vi "TR_Generate_Segmented_Plot_v5_DAQmx.vi"(0 "Settings and Parameters in":T1, 1 "Background color":u32(colorbox)=13816530, 2 "Segments Colors In":T6={"Colors array for outer segments"=[14102567, 16625249, 14742520, 7646673, 16018755, 16703632, 11262441, 4552116], "Colors array for midfield segments"=[8073876, 10935200, 34871, 12756431], "Color for central segment"=16777113, "Fill color for no segments image"=6316128}, 3 "Scale factor for outer display radius display (0.95)":dbl=0.95 format="%#_13g", 5 "Regions to mark set/selected":T4, 7 "Show magnets (T)":bool=TRUE, 9 "Show zones (T)":bool=TRUE, 11 "Error In":errorcluster) -> (4 "Settings and Parameters out":T1, 6 "Experiment Diagram":T7(plugin-control), 8 "Color to [pixel, segment, zone] correspondences":T3, 10 "Image geometrical and scaling parameters":T5, 15 "Error Out":errorcluster)   [LabVIEW 2018, in "Tracks Repair.lvlib"]
uses:
  Tracks Repair.lvlib
  SubVi's/Controls/CTL_Image_Geometrical_and_scaling_parameters.ctl
  SubVi's/Controls/CTL_Pixel_to_Zone_array.ctl
  SubVi's/Controls/CTL_Settings_cluster.ctl
  SubVi's/Controls/CTL_Histogram_parameters.ctl
  SubVi's/Controls/CTL_Filter_selector.ctl
  SubVi's/Controls/CTL_Acquisition_speed_selector.ctl
  SubVi's/Controls/CTL_Segmented_plot_parameters.ctl
  SubVi's/Controls/CTL_IO_params_cluster.ctl
  SubVi's/Controls/CTL_Conditions_Array.ctl
  SubVi's/Controls/CTL_Conditions_Cluster.ctl
  SubVi's/Controls/CTL_Condition_type.ctl
  SubVi's/Controls/CTL_Comparison_type.ctl
  SubVi's/Controls/CTL_Validity_check_criteria.ctl
  SubVi's/Controls/CTL_Response_info.ctl
  SubVi's/Controls/CTL_Condition_response_type.ctl
  SubVi's/Controls/CTL_Reponse_port_info.ctl
  SubVi's/Controls/CTL_Calibration_parameters.ctl
  SubVi's/Controls/CTL_Dispenser_calibration_info.ctl
  SubVi's/Controls/CTL_Post-processing_params.ctl
  SubVi's/Controls/CTL_Mouse_Draw_Params.ctl
  <vilib>/vision/Image Controls.llb/IMAQ Image.ctl
  Tracker.lvlib
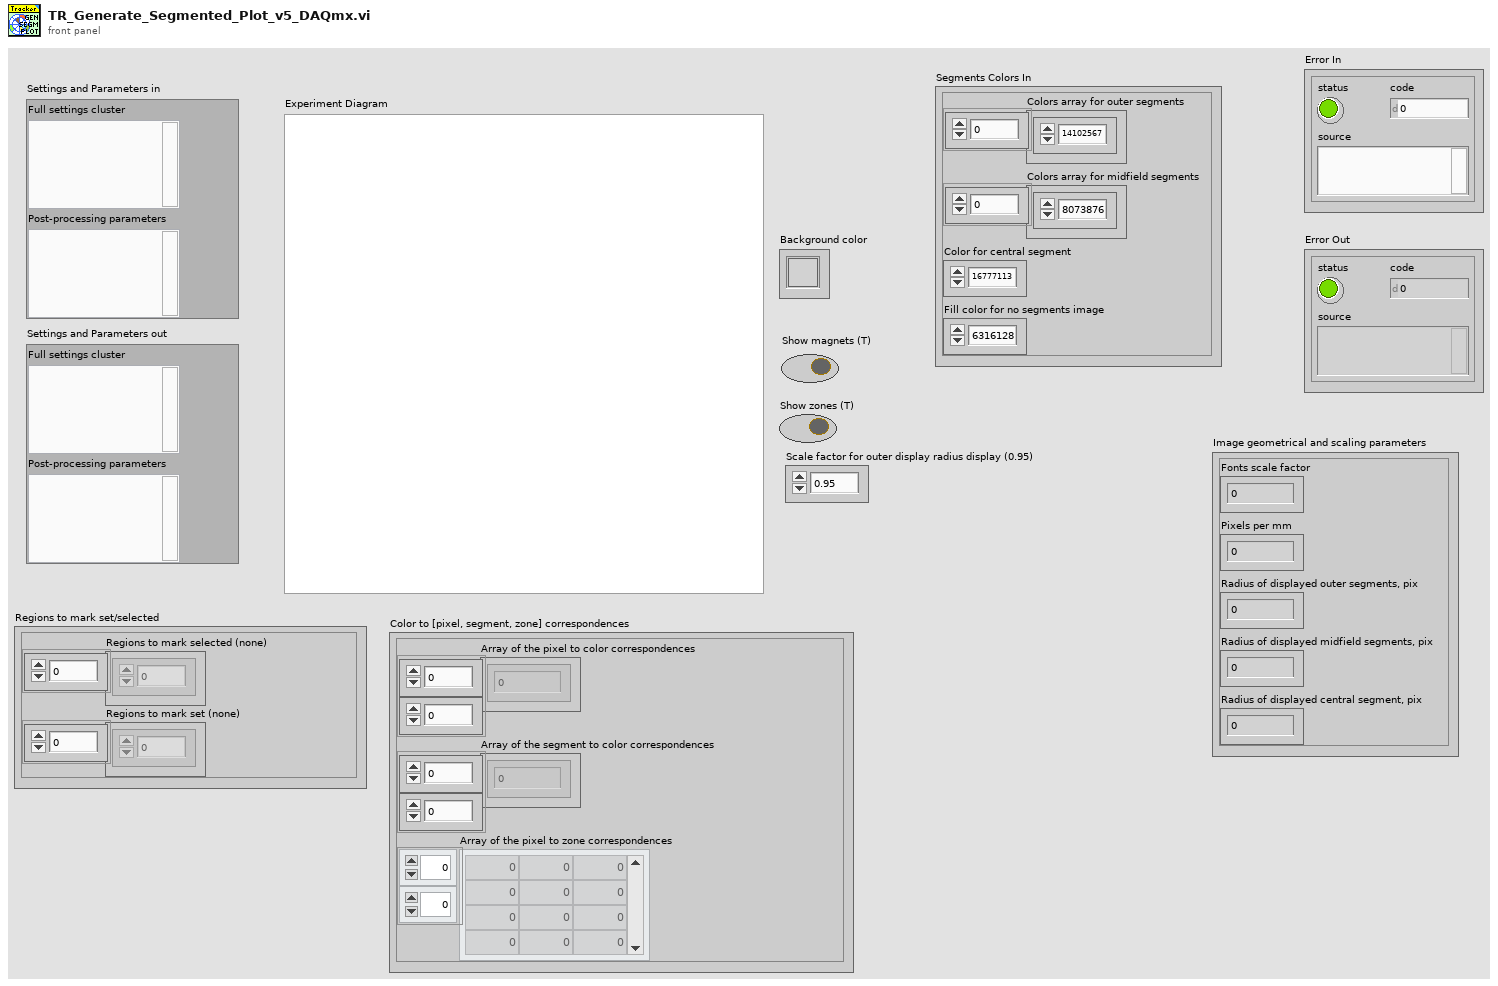
[diagram p1: front panel]
types:
  T1 = cluster{"Full settings cluster":variant, "Post-processing parameters":variant}
  T2 = typedef "Tracker.lvlib/CTL_Pixel_to_Zone_array.ctl" = i8[][]
  T3 = cluster{"Array of the pixel to color correspondences":u32[][], "Array of the segment to color correspondences":u32[][], "Array of the pixel to zone correspondences":T2}
  T4 = cluster{"Regions to mark selected (none)":u16[], "Regions to mark set (none)":u16[]}
  T5 = typedef "Tracker.lvlib/CTL_Image_Geometrical_and_scaling_parameters.ctl" = cluster{"Fonts scale factor":dbl, "Pixels per mm":dbl, "Radius of displayed outer segments, pix":dbl, "Radius of displayed midfield segments, pix":dbl, "Radius of displayed central segment, pix":dbl}
  T6 = cluster{"Colors array for outer segments":u32[], "Colors array for midfield segments":u32[], "Color for central segment":u32, "Fill color for no segments image":u32}
  T7 = typedef "IMAQ Image.ctl" = refnum<image>
  T8 = typedef "Tracker.lvlib/CTL_Post-processing_params.ctl" = cluster{"Defragment TDMS? (F)":bool, "Start time (SW)":timestamp, "Start time (HW)":u32, "Data filtering":T9, "Mouse drawing parameters":T10, "Size of the image (480x480)":cluster{"Numeric Control":dbl, "Numeric Control":dbl}, "Image ref. in":T7, "Calibration parameters":T11, "Pixel to zone":T2}
  T9 = typedef "Tracker.lvlib/CTL_Filter_selector.ctl" = cluster{"Filter type":enum16{"None", "Savitzky-Golay"}, "Length":i32, "Order":i32}
  T10 = typedef "Tracker.lvlib/CTL_Mouse_Draw_Params.ctl" = cluster{"Trace length, samples":u16, "Rainbow track":bool, "Rainbow track is speed":bool, "Bright mouse lineout":bool, "Colors array":u32[], "Pixels per mm":dbl}
  T11 = typedef "Tracker.lvlib/CTL_Calibration_parameters.ctl" = cluster{"Timing calibration sw/hw":dbl, "True FPS":dbl, "True frame time, s":dbl, "Disp. calibration info":T12}
  T12 = typedef "Tracker.lvlib/CTL_Dispenser_calibration_info.ctl" = cluster{"Channel":u8, "Speed, µl per ms":dbl}[]
  T13 = typedef "Tracker.lvlib/CTL_Settings_cluster.ctl" = cluster{"Defaults":cluster{"Default User":dbl, "VISA Resource Name ":string, "Histogram parameters":T14}, "Recording and saving":cluster{"Researcher name":string, "Name prefix":string, "Data post-processing":T9, "Stop at":dbl, "\"Stop at\" enabled":bool, "Default save folder path":path, "Acquisition FPS":T15}, "Geometry":T16, "IO parameters":T17, "Conditions presets array":T18, "Calibration parameters":T11, "Settings loaded OK":bool}
  T14 = typedef "Tracker.lvlib/CTL_Histogram_parameters.ctl" = cluster{"max":dbl, "min":dbl, "# bins":i32, "threshold":dbl, "thr. type":enum16{"higher accepted", "lower accepted"}}
  T15 = typedef "Tracker.lvlib/CTL_Acquisition_speed_selector.ctl" = enum16{"Max", "Optimal", "Eco"}
  T16 = typedef "Tracker.lvlib/CTL_Segmented_plot_parameters.ctl" = cluster{"Cage diameter, mm":u16, "Starting angle MIDFIELD":i16, "Starting angle BORDER":i16, "Radius, mm CENTER":u16, "Radius, mm MIDFIELD":u16, "N segments MIDFIELD":u8, "N segments BORDER":u8, "R-gap, mm":sgl, "Bridge swap":bool, "Bridge H. offset":sgl, "Bridge V. offset":sgl, "Twisted neck":bool, "Alt. magn. orientation":bool, "Sensor board size":enum16{"Small", "Large"}}
  T17 = typedef "Tracker.lvlib/CTL_IO_params_cluster.ctl" = cluster{"IO general config.":u16, "IO 1 configuration":u16, "IO 2 configuration":u16, "IO 3 configuration":u16, "IO 4 configuration":u16, "Activate ext. RS-232":u16, "IO inversion config.":u16, "Sync capability":u8}
  T18 = typedef "Tracker.lvlib/CTL_Conditions_Array.ctl" = T19[]
  T19 = typedef "Tracker.lvlib/CTL_Conditions_Cluster.ctl" = cluster{"Enabled":bool, "Name":string, "Specifier(s)":cluster{"Specifier enabled":bool, "Condition type":T20, "Comparison type":T21, "Value":dbl, "Validity criteria(s)":cluster{"V. check enabled":bool, "Criteria":T22, "Validity value":dbl}[]}[], "Response":T23, "Has been set":bool}
  T20 = typedef "Tracker.lvlib/CTL_Condition_type.ctl" = enum16{"Speed", "Zone", "Angle to wall"}
  T21 = typedef "Tracker.lvlib/CTL_Comparison_type.ctl" = enum16{"Less", "Less or Equal", "Equal", "Greater or Equal", "Greater", "Not Equal"}
  T22 = typedef "Tracker.lvlib/CTL_Validity_check_criteria.ctl" = enum16{"Running bout (seconds)", "Running bout (meters)"}
  T23 = typedef "Tracker.lvlib/CTL_Response_info.ctl" = cluster{"Response type":T24, "TTL port":T25, "TTL pulse length, ms":dbl}
  T24 = typedef "Tracker.lvlib/CTL_Condition_response_type.ctl" = enum16{"None", "Air puff", "Liquid reward"}
  T25 = typedef "Tracker.lvlib/CTL_Reponse_port_info.ctl" = enum16{"Port 1", "Port 2", "Port 3", "Port 4"}
  T26 = cluster{"Numeric Control":dbl, "Numeric Control":dbl}
  T27 = typedef "Tracker.lvlib/CTL_Bounding_Rectangle_of_Segments.ctl" = cluster{"Bounding rectangle for outer segments, pix":cluster{"TL W, pix":i32, "TL H, pix":i32, "RB W, pix":i32, "RB H, pix":i32}, "Bounding rectangle of the midfield segments, pix":cluster{"TL W, pix":i32, "TL H, pix":i32, "RB W, pix":i32, "RB H, pix":i32}, "Coordinates of the center of the image, pix":cluster{"W, pix":i32, "H, pix":i32}, "Bounding rectangle of the central segment, pix":cluster{"Numeric Control":i32, "Numeric Control":i32, "Numeric Control":i32, "Numeric Control":i32}}
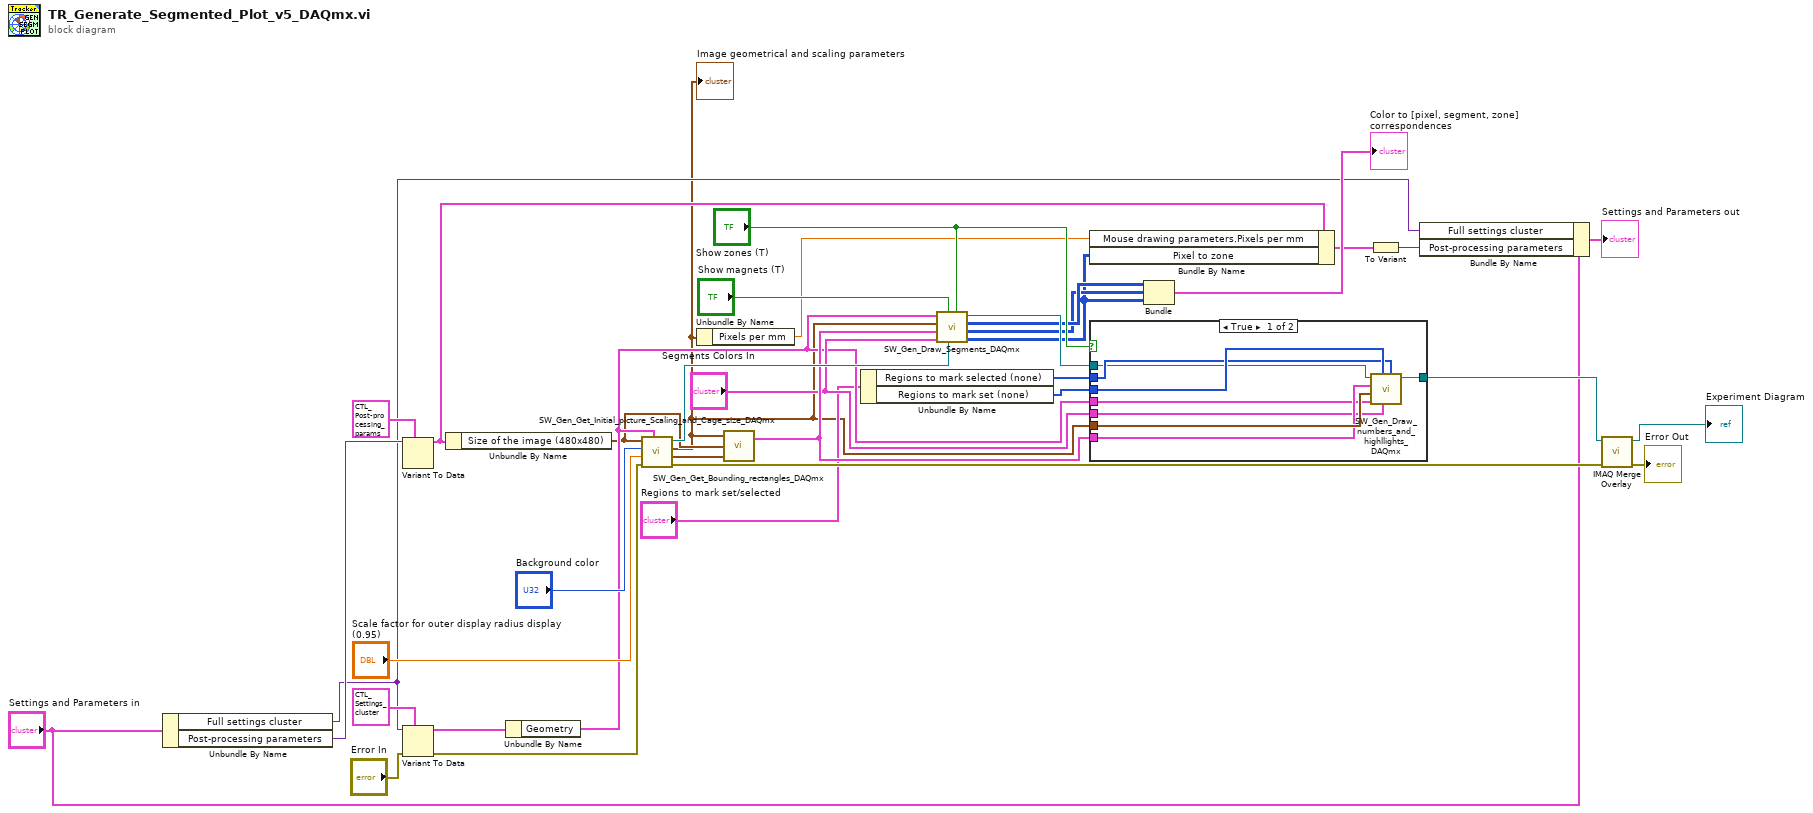
[diagram p0: block diagram]
diagram:
  n1 = Unbundle By Name("Settings and Parameters in") -> ("Full settings cluster"=w4:variant, "Post-processing parameters"=w11:variant)
  n2 = Variant To Data(type=T8 {"Defragment TDMS? (F)"=FALSE, "Start time (SW)"=timestamp(0 s since 1904-01-01), "Start time (HW)"=0, "Data filtering"={"Filter type"=enum."Savitzky-Golay", "Length"=41, "Order"=3}, "Mouse drawing parameters"={"Trace length, samples"=0, "Rainbow track"=FALSE, "Rainbow track is speed"=FALSE, "Bright mouse lineout"=FALSE, "Colors array"=[], "Pixels per mm"=0.0}, "Size of the image (480x480)"={"Numeric Control"=480.0, "Numeric Control"=480.0}, "Image ref. in"=refnum, "Calibration parameters"={"Timing calibration sw/hw"=1.0, "True FPS"=80.0, "True frame time, s"=0.0125, "Disp. calibration info"=[]}, "Pixel to zone"=[]} ("Processing parameters"), Variant=w11) -> (data=w10:T8)  [unwired: 1 in, 1 out]
  n3 = Variant To Data(error in="Error In", type=T13 {"Defaults"={"Default User"=0.0, "VISA Resource Name "="", "Histogram parameters"={"max"=300.0, "min"=0.0, "# bins"=10, "threshold"=8.0, "thr. type"=enum."higher accepted"}}, "Recording and saving"={"Researcher name"="", "Name prefix"="", "Data post-processing"={"Filter type"=enum."None", "Length"=0, "Order"=0}, "Stop at"=0.0, "\"Stop at\" enabled"=FALSE, "Default save folder path"=path "", "Acquisition FPS"=enum."Max"}, "Geometry"={"Cage diameter, mm"=0, "Starting angle MIDFIELD"=0, "Starting angle BORDER"=0, "Radius, mm CENTER"=0, "Radius, mm MIDFIELD"=0, "N segments MIDFIELD"=0, "N segments BORDER"=0, "R-gap, mm"=0.0, "Bridge swap"=FALSE, "Bridge H. offset"=0.0, "Bridge V. offset"=0.0, "Twisted neck"=FALSE, "Alt. magn. orientation"=FALSE, "Sensor board size"=enum."Small"}, "IO parameters"={"IO general config."=0, "IO 1 configuration"=0, "IO 2 configuration"=0, "IO 3 configuration"=0, "IO 4 configuration"=0, "Activate ext. RS-232"=0, "IO inversion config."=0, "Sync capability"=0}, "Conditions presets array"=[], "Calibration parameters"={"Timing calibration sw/hw"=0.0, "True FPS"=0.0, "True frame time, s"=0.0, "Disp. calibration info"=[]}, "Settings loaded OK"=FALSE} ("Settings cluster"), Variant=w4) -> (data=w23:T13, error out=w21:errorcluster)
  n4 = Unbundle By Name(w10) -> ("Size of the image (480x480)"=w9:T26)
  n5 = Unbundle By Name(w23) -> ("Geometry"=w25:T16)
  n6 = call "SW_Gen_Get_Initial_picture_Scaling_and_Cage_size_DAQmx.vi"("Input cluster of parameters"=w25, "Error In"=w21, "Scale factor for outer display radius display"="Scale factor for outer display radius display (0.95)", "Background color"="Background color", "Draw Area Size"=w9) -> ("Error Out"=w20:errorcluster, "Width of the borders combined out"=w33:cluster{"Width":i32, "Height":i32}, "Image geometrical and scaling parameters"=w2:T5, "Background Image"=w32:T7)  [unwired: 3 in]
  "Image geometrical and scaling parameters" <- w2
  n7 = Unbundle By Name(w2) -> ("Pixels per mm"=w1:dbl)
  n8 = call "SW_Gen_Get_Bounding_rectangles_DAQmx.vi"("Width of the borders combined"=w33, "Draw Area Size"=w9, "Image geometrical and scaling parameters"=w2) -> ("Bounding rectangles"=w31:T27)  [unwired: 1 in]
  n9 = Unbundle By Name("Regions to mark set/selected") -> ("Regions to mark selected (none)"=w16:u16[], "Regions to mark set (none)"=w17:u16[])
  n10 = call "SW_Gen_Draw_Segments_DAQmx.vi"("Show zones"="Show zones (T)", "Cage Image ref"=w32, "Show magnets"="Show magnets (T)", "Colors cluster"="Segments Colors In", "Bounding rectangles"=w31, "Image geometrical and scaling parameters"=w2, "Input cluster of parameters"=w25) -> ("Array of the pixel to zone correspondences"=w8:T2, "Array of the segment to color correspondences"=w14:u32[][], "Array of the pixel to color correspondences"=w15:u32[][], "Cage Image out"=w29:T7)  [unwired: 1 in]
  n11 = Bundle By Name(cluster=w10, "Mouse drawing parameters.Pixels per mm"=w1, "Pixel to zone"=w8) -> (w7:T8)
  n12 = case shown="True" "Show zones (T)" {
    tunnel: w17 -> [w44 _]
    tunnel: w16 -> [w43 _]
    tunnel: w2 -> [w42 _]
    tunnel: w31 -> [w41 _]
    tunnel: "Segments Colors In" -> [w40 _]
    tunnel: w25 -> [w39 _]
    tunnel: w29 -> [w38 w45]
    tunnel: [w37 w45] -> w26
    frame True {
      n13 = call "SW_Gen_Draw_numbers_and_highllights_DAQmx.vi"("Regions to mark selected"=w43, "Colors cluster"=w40, "Regions to mark set"=w44, "Input cluster of parameters"=w39, "Image geometrical and scaling parameters"=w42, "Bounding rectangles"=w41, "Experiment Diagram"=w38) -> ("Experiment Diagram out"=w37:T7)  [unwired: 4 in]
    }
    frame False {
    }
  }
  n14 = Bundle("Array of the pixel to color correspondences"=w15, "Array of the segment to color correspondences"=w14, "Array of the pixel to zone correspondences"=w8) -> (→"Color to [pixel, segment, zone] correspondences":T3)  [unwired: 1 in]
  n15 = To Variant(anything=w7) -> (Variant=w5:variant)
  n16 = Bundle By Name(cluster="Settings and Parameters in", "Full settings cluster"=w4, "Post-processing parameters"=w5) -> (→"Settings and Parameters out":T1)
  n17 = call "IMAQ Merge Overlay"("error in (no error)"=w20, "Image Src"=w26) -> ("error out"=→"Error Out":errorcluster, "Image Dst Out"=→"Experiment Diagram":T7)  [unwired: 8 in]
